vi "Register Control.vi"(8 "error in (no error)":errorcluster, 10 "Control to Register":refnum<vi>, 11 "SlideEngine.lvclass In":refnum<class "SlideEngine.lvclass">) -> (0 "error out":errorcluster, 3 "SlideEngine.lvclass Out":refnum<class "SlideEngine.lvclass">)   [LabVIEW 2011, in "SlideEngine.lvclass"]
doc: "This VI registers a control with the SlideEngine which will create an ActionQueue and a Consumer Daemon that is unique to that particular control.\n\nThe reason behind using unique queues and consumers is so that the same control cannot be simulateously opening and closing (which would cause very glitchy behavior). As each control maps to one queue then actions have to happen in order.\n\nGiving each control it's own queue allows for different controls to be moving at the same time."
uses:
  SlideEngine.lvclass
  SlideActions.ctl
  SlideEngine.lvclass/SlideEngine.ctl
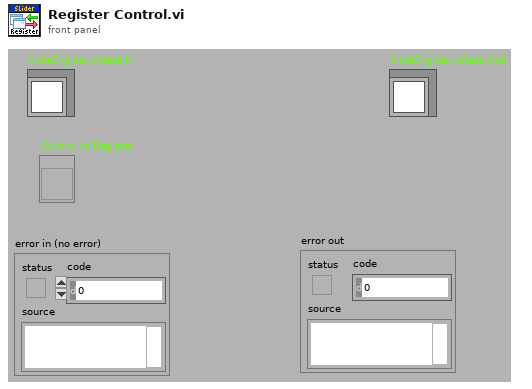
[diagram p1: front panel]
types:
  T1 = typedef "SlideActions.ctl" = enum16{"Left Open", "Left Close"}
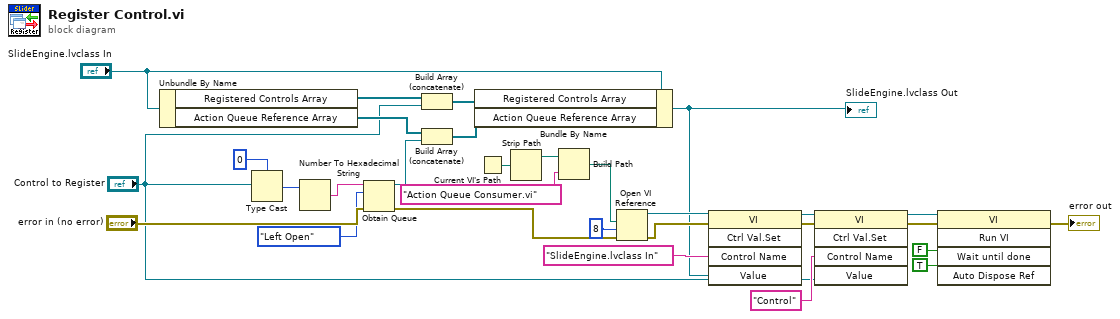
[diagram p0: block diagram]
diagram:
  n1 = Unbundle By Name("SlideEngine.lvclass In") -> ("Registered Controls Array"=w25:refnum<vi>[], "Action Queue Reference Array"=w23:refnum<queue>[])
  n2 = Type Cast(type=0, x="Control to Register") -> (*(type *) &x=w28:i32)
  n3 = Number To Hexadecimal String(2:w28) -> (0:w27:string)  [unwired: 1 out]
  n4 = Obtain Queue(name (unnamed)=w27, element data type=SlideActions."Left Open" ("Action"), error in (no error)="error in (no error)") -> (queue out=w15:refnum<queue>, error out=w14:errorcluster)  [unwired: 2 in, 1 out]
  n5 = Build Array (concatenate)(w25, "Control to Register") -> (w24:refnum<vi>[])
  n6 = Build Array (concatenate)(w23, w15) -> (w22:refnum<queue>[])
  n7 = Bundle By Name(cluster="SlideEngine.lvclass In", "Registered Controls Array"=w24, "Action Queue Reference Array"=w22) -> (w10:refnum<class "SlideEngine.lvclass">)
  "SlideEngine.lvclass Out" <- w10
  n8 = Current VI's Path() -> (path=w5:path)
  n9 = Strip Path(path=w5) -> (stripped path=w4:path)  [unwired: 1 out]
  n10 = Build Path(base path=w4, name or relative path="Action Queue Consumer.vi") -> (appended path=w2:path)
  n11 = Open VI Reference(vi path=w2, options=8, error in (no error)=w14) -> (vi reference=w21:refnum<vi>, error out=w19:errorcluster)  [unwired: 1 in, 2 out]
  n12 = invoke class="VI" method="Ctrl Val.Set"(reference=w21, error in=w19, "Control Name"="SlideEngine.lvclass In", "Value"=w10) -> (reference out=w9:refnum<vi>, error out=w20:errorcluster)  [unwired: 1 in, 3 out]
  n13 = invoke class="VI" method="Ctrl Val.Set"(reference=w9, "Control Name"="Control", "Value"="Control to Register") -> (reference out=w8:refnum<vi>)  [unwired: 2 in, 4 out]
  n14 = invoke class="VI" method="Run VI"(reference=w8, error in=w20, "Wait until done"=FALSE ("Wait Until Done"), "Auto Dispose Ref"=TRUE ("Auto Dispose Reference")) -> (error out=→"error out":errorcluster)  [unwired: 1 in, 4 out]
